vi "NCD Update Settings Setpoints.vi"(8 "error in (no error)":errorcluster, 10 "Message Data":variant, 11 "Data Cluster":T1={"MFC Definition"={"MFC Port"="", "MFC Enable"=TRUE, "Baud Rate"=0, "Interface type"=enum."RS-485", "Address"=0}, "Set Point Options"={"Setpoint Value"=0.0, "Mass Flow EU 2"="", "Setpoint Source"="", "Valve Mode"=""}, "Writer Queue"=refnum, "Enable"=FALSE, "Update Rate"=0, "MRC Chamber Enable"=FALSE, "Selected Gas"="", "Address String"=""} {"Set Point Options"."Setpoint Value" min=0.0 max=0.62495 format="%.5f"}) -> (0 "error out":errorcluster, 1 "Status":string, 2 "Send Resp":bool, 3 "Data Cluster out":T1={"MFC Definition"={"MFC Port"="", "MFC Enable"=TRUE, "Baud Rate"=0, "Interface type"=enum."RS-485", "Address"=0}, "Set Point Options"={"Setpoint Value"=0.0, "Mass Flow EU 2"="", "Setpoint Source"="", "Valve Mode"=""}, "Writer Queue"=refnum, "Enable"=FALSE, "Update Rate"=0, "MRC Chamber Enable"=FALSE, "Selected Gas"="", "Address String"=""} {"Set Point Options"."Setpoint Value" min=0.0 max=0.62495 format="%.5f"})   [LabVIEW 2020, in "MRC Module.lvlib"]
uses:
  MRC Module.lvlib
  MRC Configuration.ctl
  support/Message Queue/Message Cluster.ctl
  support/HW Message Cluster.ctl
  support/Message Queue/Message Queue.lvlib
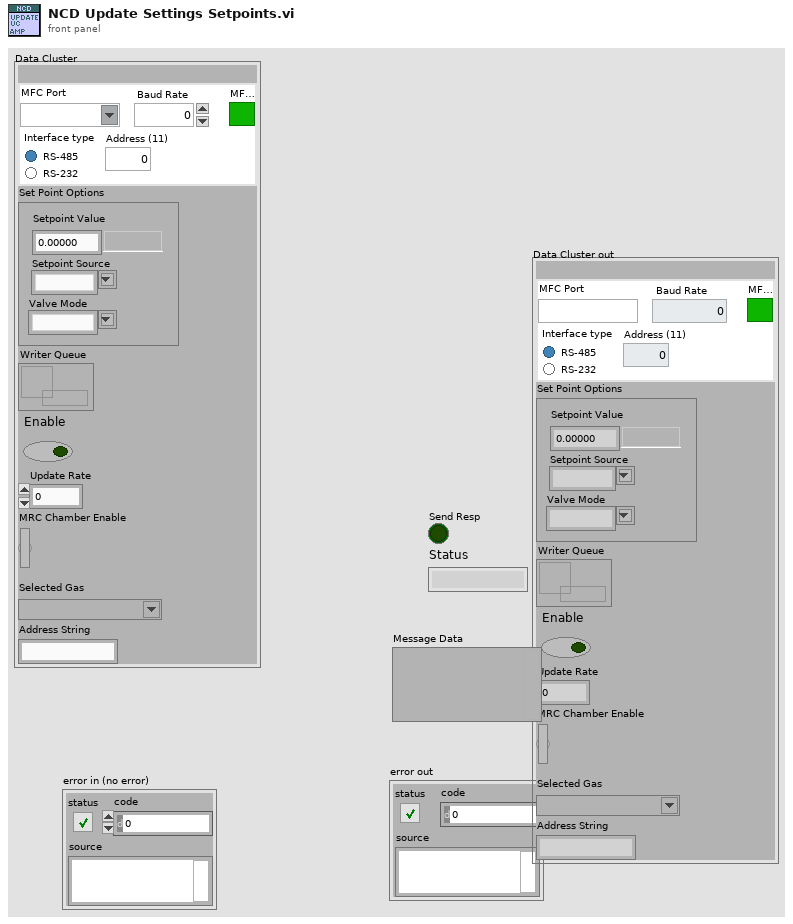
[diagram p1: front panel]
types:
  T1 = typedef "MRC Module.lvlib/MRC Configuration.ctl" = cluster{"MFC Definition":cluster{"MFC Port":refnum<visa-resource-name>, "MFC Enable":bool, "Baud Rate":i32, "Interface type":enum32{"RS-485", "RS-232"}, "Address":i32}, "Set Point Options":cluster{"Setpoint Value":dbl, "Mass Flow EU 2":string, "Setpoint Source":string, "Valve Mode":string}, "Writer Queue":refnum<queue>, "Enable":bool, "Update Rate":u32, "MRC Chamber Enable":bool, "Selected Gas":string, "Address String":string}
  T2 = typedef "Message Queue.lvlib/HW Message Cluster.ctl" = cluster{"Writer Queue":refnum<queue>, "Writer Data":T3}
  T3 = typedef "Message Queue.lvlib/Message Cluster.ctl" = cluster{"Message":string, "Message Data":variant}
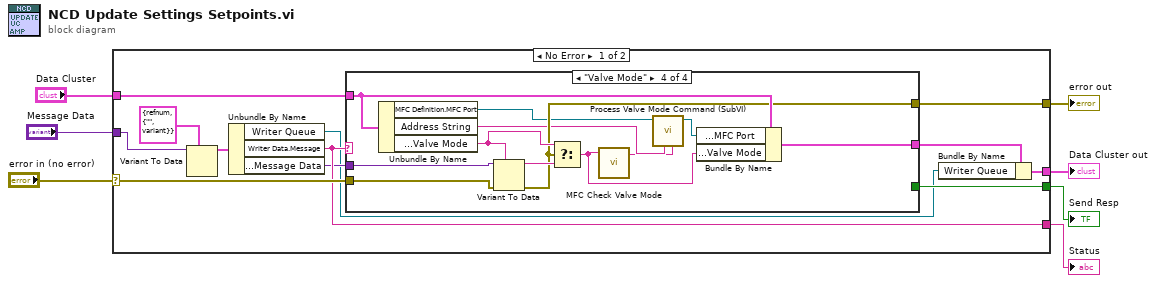
[diagram p0: block diagram]
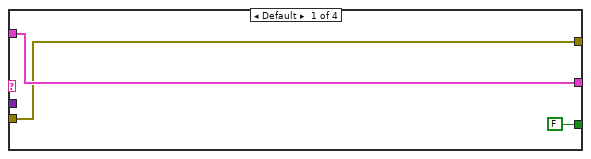
[diagram p2: hidden frame]
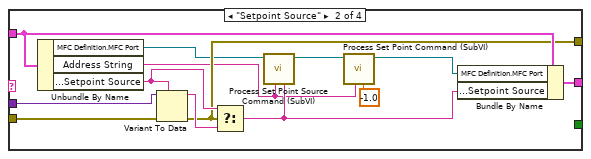
[diagram p3: hidden frame]
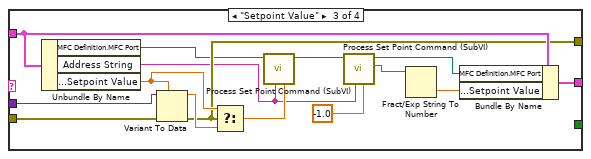
[diagram p4: hidden frame]
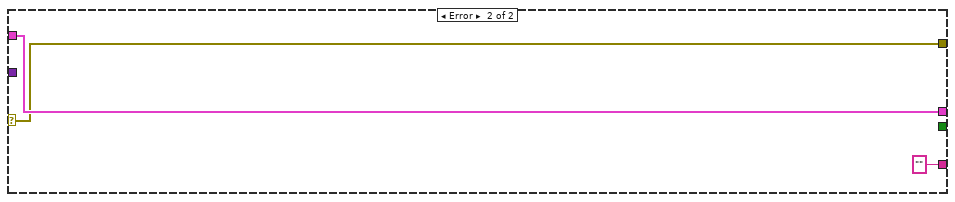
[diagram p5: hidden frame]
diagram:
  n1 = case shown="No Error" "error in (no error)" {
    selector: "error in (no error)" -> [w16 w64]
    tunnel: [w19 w64] -> w7
    tunnel: "Data Cluster" -> [w12 w65]
    tunnel: [w14 w65] -> w5
    tunnel: "Message Data" -> [w17 _]
    tunnel: [w15 _] -> w2
    tunnel: [w11 "" ("Message")] -> w1
    frame No Error {
      n2 = Variant To Data(type=T2 {"Writer Queue"=refnum, "Writer Data"={"Message"="", "Message Data"=variant}}, Variant=w17) -> (data=w13:T2)  [unwired: 1 in, 1 out]
      n3 = Unbundle By Name(w13) -> ("Writer Queue"=w8:refnum<queue>, "Writer Data.Message"=w11:string, "Writer Data.Message Data"=w10:variant)
      n4 = case shown="\"Valve Mode\"" w11 {
        tunnel: w10 -> [_ w34 w49 w61]
        tunnel: [w22 w33 w48 w60] -> w18
        tunnel: w12 -> [w22 w35 w50 w62]
        tunnel: w16 -> [w21 w30 w45 w57]
        tunnel: [w21 w29 w44 w56] -> w19
        tunnel: [FALSE ("Send Resp") _ _ _] -> w15
        frame Default {
        }
        frame "Setpoint Source" {
          n5 = Unbundle By Name(w35) -> ("MFC Definition.MFC Port"=w28:refnum<visa-resource-name>, "Address String"=w25:string, "Set Point Options.Setpoint Source"=w32:string)
          n6 = Variant To Data(error in=w30, type=w32, Variant=w34) -> (data=w31:string, error out=w29:errorcluster)
          n7 = Select(t=w32, s=w29, f=w31) -> (s? t:f=w27:string)
          n8 = call "Process Set Point Source Command (SubVI).vi"("Set Point Source In"=w27, "Address"=w25, "VISA Refnum in"=w28) -> ("VISA Refnum out"=w26:refnum<visa-resource-name>)  [unwired: 6 in, 2 out]
          n9 = call "Process Set Point Command (SubVI).vi"("Setpoint"=-1.0, "Address"=w25, "VISA Refnum in"=w26) -> ("VISA Refnum out"=w23:refnum<visa-resource-name>)  [unwired: 6 in, 2 out]
          n10 = Bundle By Name(cluster=w35, "MFC Definition.MFC Port"=w23, "Set Point Options.Setpoint Source"=w27) -> (w33:T1)
        }
        frame "Setpoint Value" {
          n11 = Unbundle By Name(w50) -> ("MFC Definition.MFC Port"=w43:refnum<visa-resource-name>, "Address String"=w39:string, "Set Point Options.Setpoint Value"=w47:dbl)
          n12 = Variant To Data(error in=w45, type=w47, Variant=w49) -> (data=w46:dbl, error out=w44:errorcluster)
          n13 = Select(t=w47, s=w44, f=w46) -> (s? t:f=w42:dbl)
          n14 = call "Process Set Point Command (SubVI).vi"("Setpoint"=w42, "Address"=w39, "VISA Refnum in"=w43) -> ("VISA Refnum out"=w41:refnum<visa-resource-name>)  [unwired: 6 in, 2 out]
          n15 = call "Process Set Point Command (SubVI).vi"("Setpoint"=-1.0, "Address"=w39, "VISA Refnum in"=w41) -> ("Setpoint Value Out"=w37:string, "VISA Refnum out"=w40:refnum<visa-resource-name>)  [unwired: 6 in, 1 out]
          n16 = Fract/Exp String To Number(string=w37) -> (number=w36:dbl)  [unwired: 3 in, 1 out]
          n17 = Bundle By Name(cluster=w50, "MFC Definition.MFC Port"=w40, "Set Point Options.Setpoint Value"=w36) -> (w48:T1)
        }
        frame "Valve Mode" {
          n18 = Unbundle By Name(w62) -> ("MFC Definition.MFC Port"=w54:refnum<visa-resource-name>, "Address String"=w55:string, "Set Point Options.Valve Mode"=w59:string)
          n19 = Variant To Data(error in=w57, type=w59, Variant=w61) -> (data=w58:string, error out=w56:errorcluster)
          n20 = Select(t=w59, s=w56, f=w58) -> (s? t:f=w52:string)
          n21 = call "MFC Check Valve Mode.vi"("Valve Mode"=w52) -> ("Valve Mode out"=w51:string)  [unwired: 10 in]
          n22 = call "Process Valve Mode Command (SubVI).vi"("Valve Mode In"=w51, "Address"=w55, "VISA Refnum in"=w54) -> ("VISA Refnum out"=w53:refnum<visa-resource-name>)  [unwired: 6 in, 2 out]
          n23 = Bundle By Name(cluster=w62, "MFC Definition.MFC Port"=w53, "Set Point Options.Valve Mode"=w52) -> (w60:T1)
        }
      }
      n24 = Bundle By Name(cluster=w18, "Writer Queue"=w8) -> (w14:T1)
    }
    frame Error {
    }
  }
  "error out" <- w7
  "Data Cluster out" <- w5
  "Send Resp" <- w2
  "Status" <- w1
